vi "Get State Ctrl Refs.vi"(8 "error in (no error)":errorcluster, 11 "vi ref":refnum<vi>) -> (0 "error out":errorcluster, 3 "All Controls[]":refnum<vi>[](array[refnum]))   [LabVIEW 2021]
panel:
  out "No. of Ctrls to Save":i32
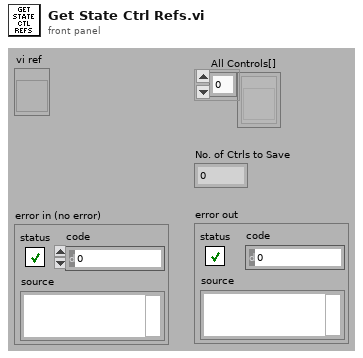
[diagram p1: front panel]
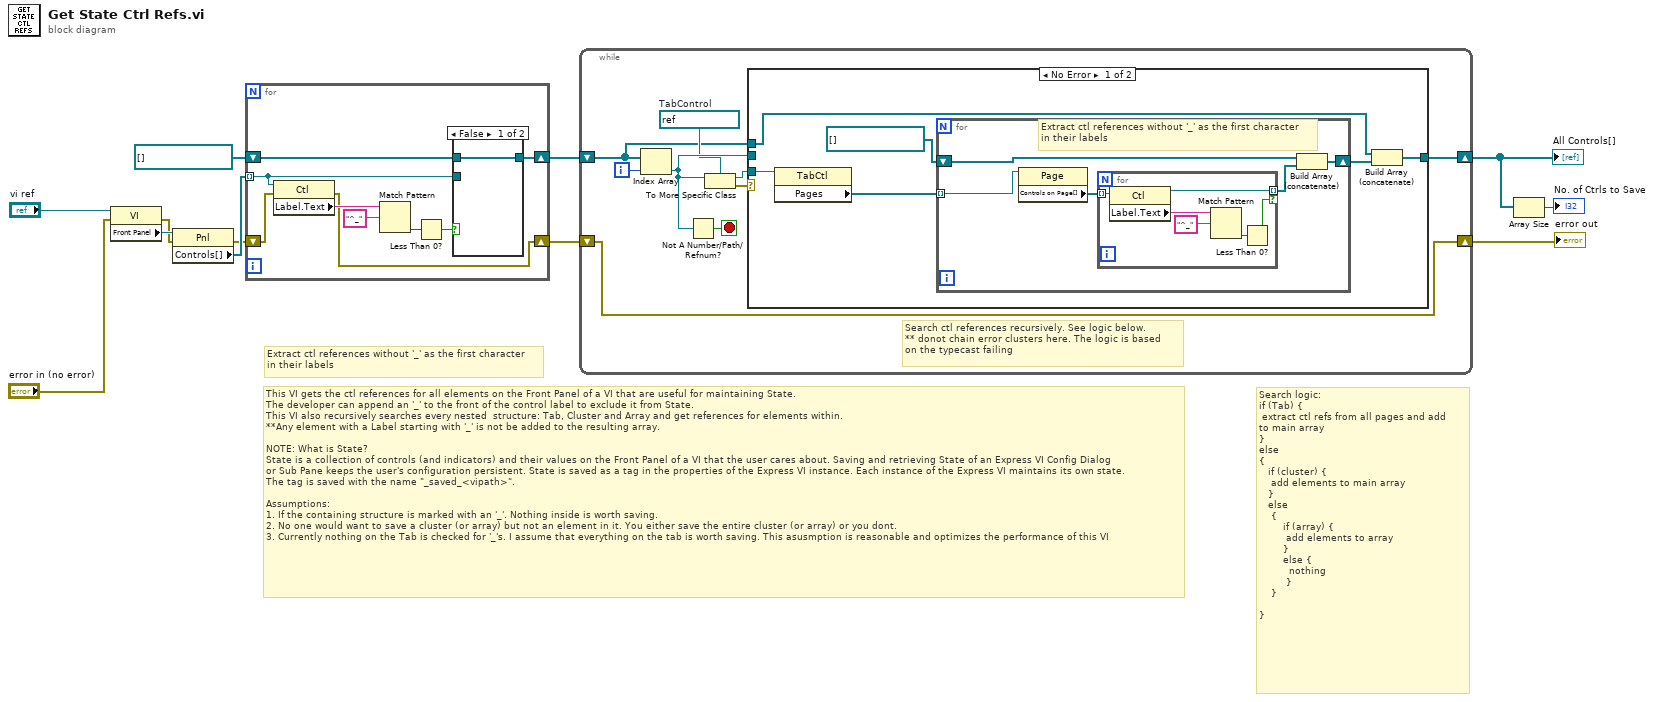
[diagram p0: block diagram]
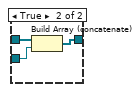
[diagram p2: hidden frame]
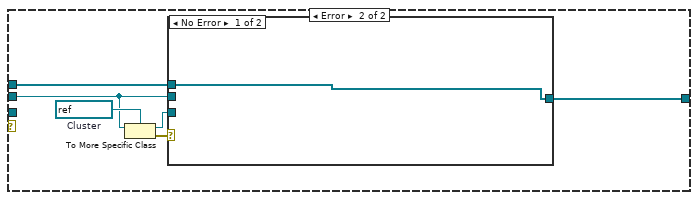
[diagram p3: hidden frame]
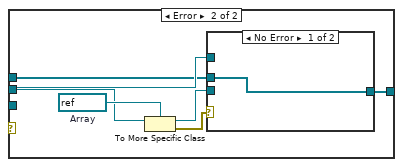
[diagram p4: hidden frame]
diagram:
  # "Search logic:\nif (Tab) {\n extract ctl refs from all pages and add         to main array\n}\nelse\n{\n   if (cluster) {\n    add elements to main array \n   }\n   else\n    {\n        if (array) {\n         add elements to array\n        }\n        else { \n          nothing\n         }    \n    }\n\n}"
  # "Extract ctl references without '_' as the first character\nin their labels"
  # "This VI gets the ctl references for all elements on the Front Panel of a VI that are useful for maintaining State. \nThe developer can append an '_' to the front of the control label to exclude it from State. \nThis VI also recursively searches every nested  structure: Tab, Cluster and Array and get references for elements within. \n**Any element with a Label starting with '_' is not be added to the resulting array.\n\nNOTE: What is State?\nState is a collection of controls (and indicators) and their values on the Front Panel of a VI that the user cares about. Saving and retrieving State of an Express VI Config Dialog \nor Sub Pane keeps the user's configuration persistent. State is saved as a tag in the properties of the Express VI instance. Each instance of the Express VI maintains its own state. \nThe tag is saved with the name \"_saved_<vipath>\". \n\nAssumptions: \n1. If the containing structure is marked with an '_'. Nothing inside is worth saving. \n2. No one would want to save a cluster (or array) but not an element in it. You either save the entire cluster (or array) or you dont.\n3. Currently nothing on the Tab is checked for '_'s. I assume that everything on the tab is worth saving. This asusmption is reasonable and optimizes the performance of this VI"
  n1 = property class="VI"(reference="vi ref", error in="error in (no error)") -> (error out=w5:errorcluster, "Front Panel"=w12:refnum<vi>)  [unwired: 1 out]
  n2 = property class="Pnl"(reference=w12, error in=w5) -> (error out=w4:errorcluster, "Controls[]"=w10:refnum<vi>[])  [unwired: 1 out]
  n3 = for {
    tunnel: w10 -> [w17] mode=indexing
    shift-right: [w15] -> w8
    shift-left: refnum<vi>[] [] -> [w16]
    shift-right: [w13] -> w2
    shift-left: w4 -> [w14]
    n4 = property class="Ctl"(reference=w17, error in=w14) -> (error out=w13:errorcluster, "Label.Text"=w21:string)  [unwired: 1 out]
    n5 = Match Pattern(string=w21, regular expression="^_") -> (offset past match=w19:i32)  [unwired: 1 in, 3 out]
    n6 = Less Than 0?(x=w19) -> (x < 0?=w18:bool)
    n7 = case shown="False" w18 {
      tunnel: w17 -> [_ w25]
      tunnel: w16 -> [w22 w24]
      tunnel: [w22 w23] -> w15
      frame False {
      }
      frame True {
        n8 = Build Array (concatenate)(w24, w25) -> (w23:refnum<vi>[])
      }
    }
  }
  n9 = while {
    shift-left: w8 -> [w28]
    shift-right: [w34] -> w7
    shift-right: [w26] -> w1
    shift-left: w2 -> [w26]
    i -> [w27]
    stop <- w33 stop-if-true
    w30 = refnum<vi> refnum  # TabControl
    # "Search ctl references recursively. See logic below.\n** donot chain error clusters here. The logic is based \non the typecast failing"
    n10 = Index Array(array=w28, index=w27) -> (element=w32:refnum<vi>)
    n11 = Not A Number/Path/Refnum?(number/path/refnum=w32) -> (NaN/Path/Refnum?=w33:bool)
    n12 = To More Specific Class(target class=w30, reference=w32) -> (specific class reference=w31:refnum<vi>, error out=w29:errorcluster)  [unwired: 1 in]
    n13 = case shown="No Error" w29 {
      tunnel: w31 -> [w40 _]
      tunnel: w32 -> [_ w54]
      tunnel: [w38 w53] -> w34
      tunnel: w28 -> [w37 w52]
      frame No Error {
        n14 = property class="TabCtl"(reference=w40) -> ("Pages"=w39:refnum<vi>[])  [unwired: 1 in, 2 out]
        n15 = for {
          tunnel: w39 -> [w45] mode=indexing
          shift-right: [w43] -> w36
          shift-left: refnum<vi>[] [] -> [w44]
          # "Extract ctl references without '_' as the first character\nin their labels"
          n16 = property class="Page"(reference=w45) -> ("Controls on Page[]"=w42:refnum<vi>[])  [unwired: 1 in, 2 out]
          n17 = for {
            tunnel: w42 -> [w48] mode=indexing
            tunnel: [w47] -> w41 mode=indexing if=w46
            n18 = property class="Ctl"(reference=w48) -> (reference out=w47:refnum<vi>, "Label.Text"=w51:string)  [unwired: 1 in, 1 out]
            n19 = Match Pattern(string=w51, regular expression="^_") -> (offset past match=w49:i32)  [unwired: 1 in, 3 out]
            n20 = Less Than 0?(x=w49) -> (x < 0?=w46:bool)
          }
          n21 = Build Array (concatenate)(w44, w41) -> (w43:refnum<vi>[])
        }
        n22 = Build Array (concatenate)(w37, w36) -> (w38:refnum<vi>[])
      }
      frame Error {
        w57 = refnum<vi> refnum  # Cluster
        n23 = To More Specific Class(target class=w57, reference=w54) -> (specific class reference=w56:refnum<vi>, error out=w55:errorcluster)  [unwired: 1 in]
        n24 = case shown="No Error" w55 {
          tunnel: w56 -> [_ _]
          tunnel: w54 -> [_ w61]
          tunnel: [w58 w60] -> w53
          tunnel: w52 -> [w58 w59]
          frame No Error {
          }
          frame Error {
            w64 = refnum<vi> refnum  # Array
            n25 = To More Specific Class(target class=w64, reference=w61) -> (specific class reference=w63:refnum<vi>, error out=w62:errorcluster)  [unwired: 1 in]
            n26 = case shown="No Error" w62 {
              tunnel: w63 -> [_ _]
              tunnel: w61 -> [_ _]
              tunnel: [w65 w66] -> w60
              tunnel: w59 -> [w65 w66]
              frame No Error {
              }
              frame Error {
              }
            }
          }
        }
      }
    }
  }
  "All Controls[]" <- w7
  "error out" <- w1
  n27 = Array Size(array=w7) -> (size(s)=→"No. of Ctrls to Save":i32)
